vi "Organise_String_Array.vi"(1 "Input Array":string[](array[string])) -> (0 "Output Array":string[](array[string]))   [LabVIEW 2021]
panel:
  in  "milliseconds to wait":u32=100
  in  "downFast":bool
  in  "upFast":bool
  out "Move Up 2":bool
  in  "OK":bool
  in  "Delete":bool
  in  "Move Down":bool
  in  "Move Up":bool
  in  "Listbox":i32[](listbox)
  # "Note you can now DRAG items to reorder the list!\n\nThe insertion point does not highlight, but so long as the control border is dotted, it is responding."
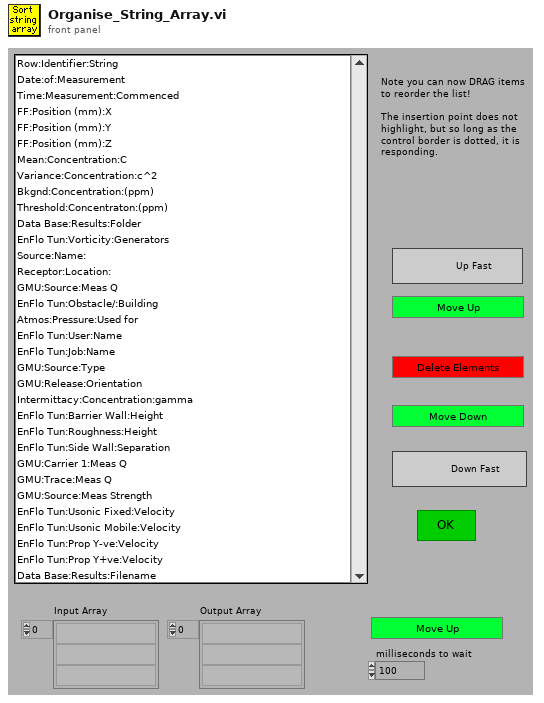
[diagram p1: front panel]
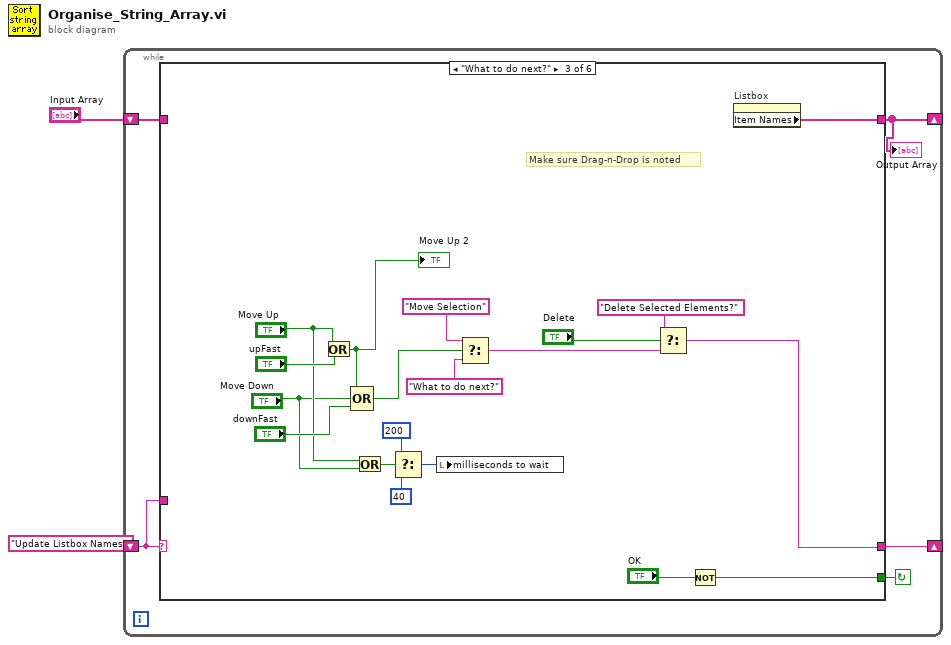
[diagram p0: block diagram]
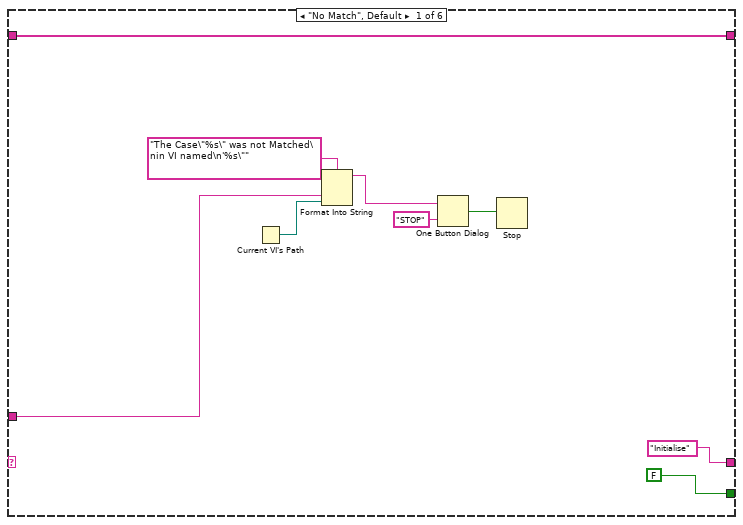
[diagram p2: hidden frame]
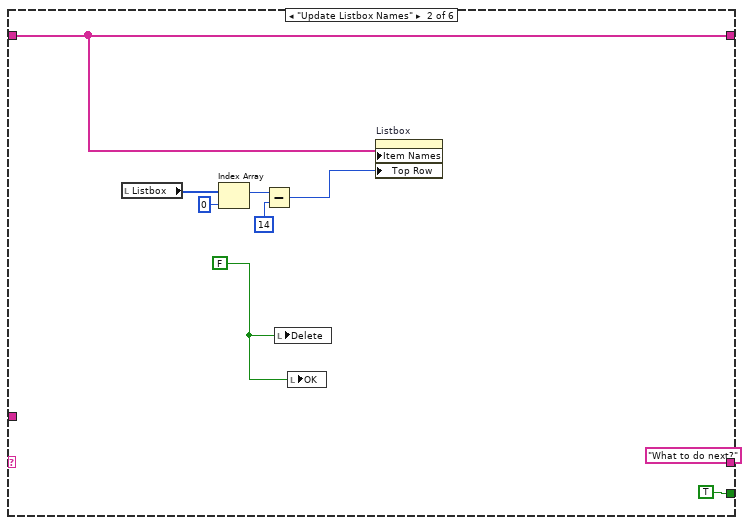
[diagram p3: hidden frame]
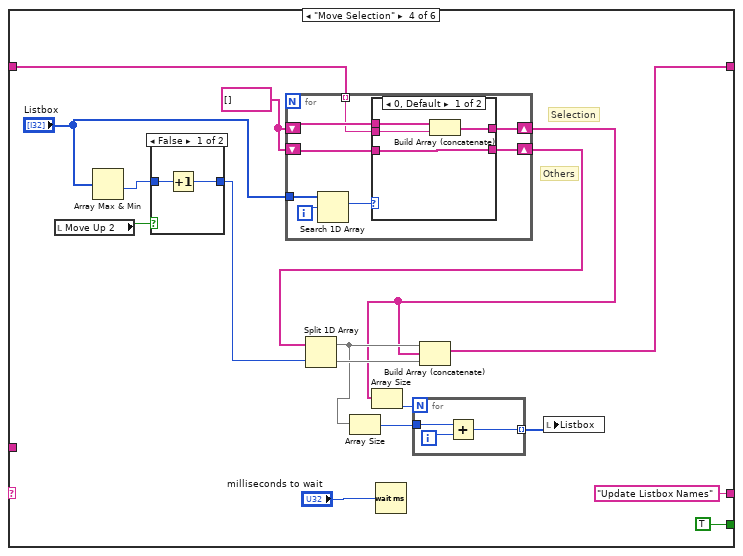
[diagram p4: hidden frame]
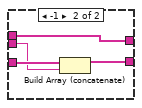
[diagram p5: hidden frame]
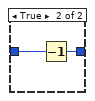
[diagram p6: hidden frame]
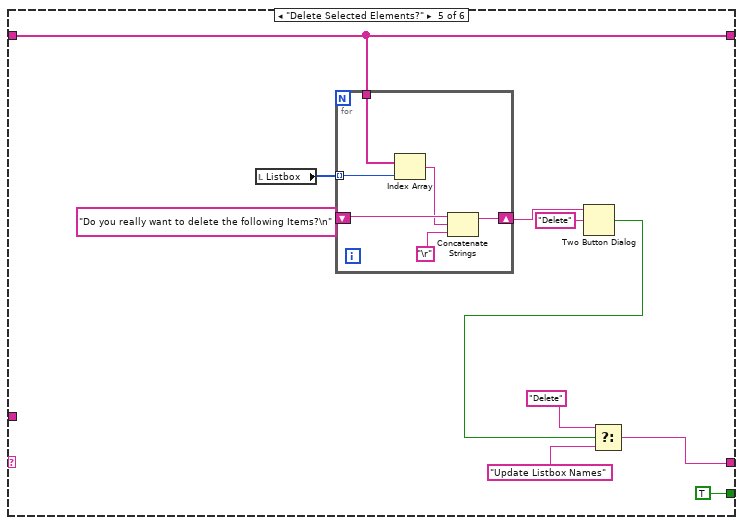
[diagram p7: hidden frame]
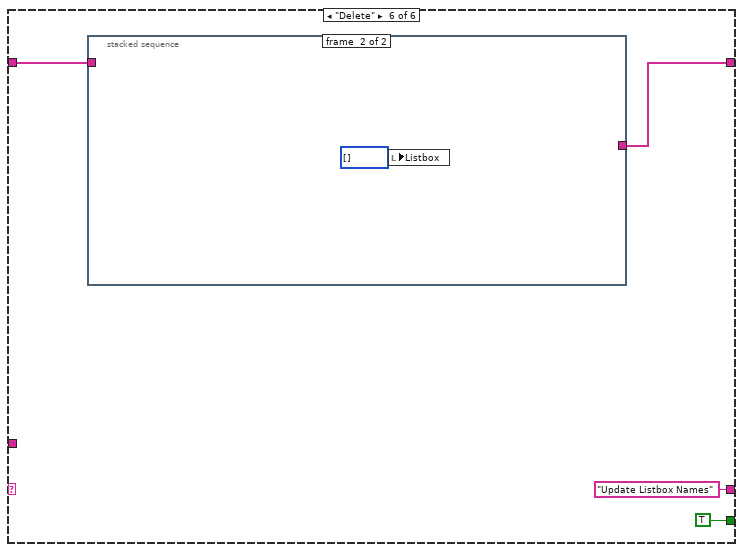
[diagram p8: hidden frame]
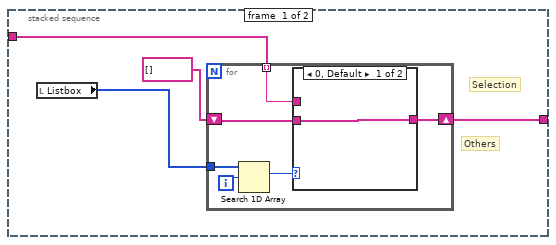
[diagram p9: hidden frame]
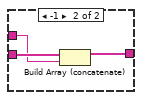
[diagram p10: hidden frame]
diagram:
  n1 = while {
    shift-left: "Input Array" -> [w4]
    shift-right: [w3] -> _
    shift-left: "Update Listbox Names" -> [w5]
    shift-right: [w6] -> _
    stop <- w7 continue-if-true
    n2 = case shown="\"What to do next?\"" w5 {
      tunnel: [FALSE TRUE w43 TRUE TRUE TRUE] -> w7
      tunnel: ["Initialise" "What to do next?" w38 "Update Listbox Names" w86 "Update Listbox Names"] -> w6
      tunnel: w5 -> [w11 _ _ _ _ _]
      tunnel: w4 -> [w8 w23 _ w55 w92 w104]
      tunnel: [w8 w23 w36 w54 w92 w101] -> w3
      frame "No Match", Default {
        n3 = Current VI's Path() -> (path=w10:path)
        n4 = Format Into String(format string="The Case\"%s\" was not Matched\nin VI named\n'%s\"" ("Format String"), w11, w10) -> (resulting string=w14:string)  [unwired: 2 in, 1 out]
        n5 = One Button Dialog(message=w14, button name ("OK")="STOP") -> (true=w12:bool)
        n6 = Stop(stop? (T)=w12) -> ()
      }
      frame "Update Listbox Names" {
        w22 = FALSE
        n7 = local read "Listbox"() -> (w18:i32[])
        n8 = Index Array(array=w18, index=0 ("Index")) -> (element=w20:i32)
        n9 = Subtract(x=w20, y=14) -> (x-y=w17:i32)
        n10 = local write "Delete"(w22) -> ()
        n11 = local write "OK"(w22) -> ()
        n12 = property on="Listbox" class="LstBox (strict)"("Item Names"=w23, "Top Row"=w17) -> ()  [unwired: 2 in, 2 out]
      }
      frame "What to do next?" {
        # "Make sure Drag-n-Drop is noted"
        n13 = Or(x="Move Up", y="upFast") -> (x .or. y?=w33:bool)
        "Move Up 2" <- w33
        n14 = Compound Arithmetic op=OR(w33, "Move Down", "downFast") -> (w32:bool)
        n15 = Or(x="Move Up", y="Move Down") -> (x .or. y?=w29:bool)
        n16 = Select(t=u32 200, s=w29, f=u32 40 ("milliseconds to wait")) -> (s? t:f=w27:u32)
        n17 = local write "milliseconds to wait"(w27) -> ()
        n18 = Select(t="Move Selection", s=w32, f="What to do next?") -> (s? t:f=w40:string)
        n19 = Select(t="Delete Selected Elements?", s="Delete", f=w40) -> (s? t:f=w38:string)
        n20 = Not(x="OK") -> (.not. x?=w43:bool)
        n21 = property on="Listbox" class="LstBox (strict)"() -> ("Item Names"=w36:string[])  [unwired: 2 in, 2 out]
      }
      frame "Move Selection" {
        w60 = string[] []
        # "Others"
        # "Selection"
        n22 = local read "Move Up 2"() -> (w61:bool)
        n23 = Array Max & Min(array="Listbox") -> (min value=w56:i32)  [unwired: 3 out]
        n24 = case shown="False" w61 {
          tunnel: w56 -> [w82 w84]
          tunnel: [w81 w83] -> w53
          frame False {
            n25 = Increment(x=w82) -> (x+1=w81:i32)
          }
          frame True {
            n26 = Decrement(x=w84) -> (x-1=w83:i32)
          }
        }
        n27 = for {
          tunnel: "Listbox" -> [w71]
          shift-right: [w67] -> w50
          shift-left: w60 -> [w69]
          shift-right: [w65] -> w59
          shift-left: w60 -> [w66]
          tunnel: w55 -> [w68] mode=indexing
          i -> [w72]
          n28 = Search 1D Array(1D array=w71, element=w72) -> (index of element=w70:i32)  [unwired: 1 out]
          n29 = case shown="0, Default" w70 {
            tunnel: w69 -> [w76 w78]
            tunnel: w68 -> [w75 w79]
            tunnel: [w74 w78] -> w67
            tunnel: w66 -> [w73 w80]
            tunnel: [w73 w77] -> w65
            frame 0, Default {
              n30 = Build Array (concatenate)(w76, w75) -> (w74:string[])
            }
            frame -1 {
              n31 = Build Array (concatenate)(w80, w79) -> (w77:string[])
            }
          }
        }
        n32 = Split 1D Array(array=w59, index=w53) -> (first subarray=w52:string[], second subarray=w58:string[])
        n33 = Array Size(array=w52) -> (size(s)=w51:i32)
        n34 = Array Size(array=w50) -> (size(s)=w49:i32)
        n35 = Wait (ms)(milliseconds to wait="milliseconds to wait") -> ()  [unwired: 1 out]
        n36 = for {
          N: w49 -> [_]
          tunnel: w51 -> [w63]
          tunnel: [w62] -> w46 mode=indexing
          i -> [w64]
          n37 = Add(x=w63, y=w64) -> (x+y=w62:i32)
        }
        n38 = Build Array (concatenate)(w52, w50, w58) -> (w54:string[])
        n39 = local write "Listbox"(w46) -> ()
      }
      frame "Delete Selected Elements?" {
        n40 = local read "Listbox"() -> (w93:i32[])
        n41 = for {
          tunnel: w93 -> [w100] mode=indexing
          tunnel: w92 -> [w99]
          shift-right: [w95] -> w90
          shift-left: "Do you really want to delete the following Items?\n" -> [w98]
          n42 = Index Array(array=w99, index=w100) -> (element=w96:string)
          n43 = Concatenate Strings(w98, w96, "\r") -> (w95:string)
        }
        n44 = Two Button Dialog(message=w90, 2:"Delete" ("T button name (\"OK\")")) -> (T button?=w89:bool)  [unwired: 1 out]
        n45 = Select(t="Delete", s=w89, f="Update Listbox Names") -> (s? t:f=w86:string)
      }
      frame "Delete" {
        n46 = stacked-sequence {
          tunnel: w104 -> [w107 _]
          tunnel: [w105 _] -> w101
          frame #0 {
            # "Others"
            # "Selection"
            n47 = local read "Listbox"() -> (w106:i32[])
            n48 = for {
              tunnel: w106 -> [w113]
              shift-right: [w109] -> w105
              shift-left: string[] [] -> [w110]
              tunnel: w107 -> [w111] mode=indexing
              i -> [w114]
              n49 = Search 1D Array(1D array=w113, element=w114) -> (index of element=w112:i32)  [unwired: 1 out]
              n50 = case shown="0, Default" w112 {
                tunnel: w111 -> [_ w117]
                tunnel: w110 -> [w115 w118]
                tunnel: [w115 w116] -> w109
                frame 0, Default {
                }
                frame -1 {
                  n51 = Build Array (concatenate)(w118, w117) -> (w116:string[])
                }
              }
            }
          }
          frame #1 {
            n52 = local write "Listbox"(i32[] [] ("Listbox")) -> ()
          }
        }
      }
    }
    "Output Array" <- w3
  }
